vi "Read From String.vi"(8 "error in (no error)":errorcluster, 11 "JSON string":string) -> (0 "error out":errorcluster, 3 "input settings":T1={"PDM clock rate"=51200.0, "decimation factor"=1, "bit clock direction"=enum."In", "logic level"=enum."3.3 V"} {"decimation factor" items=["24"=24, "32"=32, "48"=48, "64"=64, "96"=96, "128"=128]; "PDM clock rate" format="%#_6p"})   [LabVIEW 2022 SP3, in "PDM input cfg file.lvlib"]
uses:
  PDM input cfg file.lvlib
  controls/PDM/PDM input settings.ctl
  <vilib>/PDM Acquisition Toolkit/shared/controls/decimation order.ctl
  controls/bit clock direction.ctl
  <vilib>/PDM Acquisition Toolkit/host/Classes/Session/Controls/Logic Levels.ctl
  controls/PDM/PDM input settings_json.ctl
  <vilib>/PDM Acquisition Toolkit/shared/PDM Shared.lvlib
  <vilib>/PDM Acquisition Toolkit/host/Classes/Session/DecoderSession.lvclass
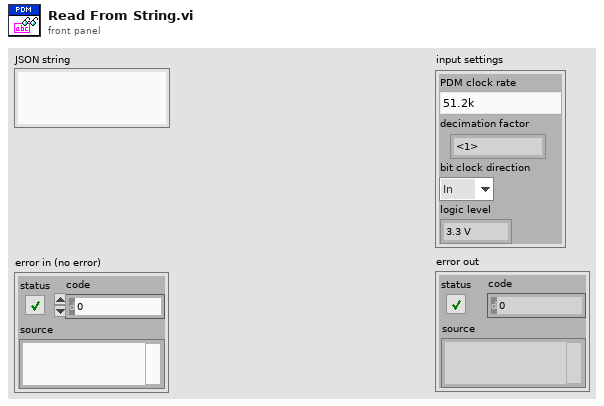
[diagram p1: front panel]
types:
  T1 = typedef "PDM input settings.ctl" = cluster{"PDM clock rate":dbl, "decimation factor":T2, "bit clock direction":T3, "logic level":T4}
  T2 = typedef "PDM Shared.lvlib/decimation order.ctl" = u16
  T3 = typedef "bit clock direction.ctl" = enum32{"In", "Out"}
  T4 = typedef "PDM Acquisition Class Library.lvlib/DecoderSession.lvclass/Logic Levels.ctl" = enum16{"3.3 V", "1.8 V", "1.2 V"}
  T5 = typedef "PDM input settings_json.ctl" = cluster{"PDM clock rate":dbl, "decimation factor":dbl, "bit clock direction":string, "logic level":string}
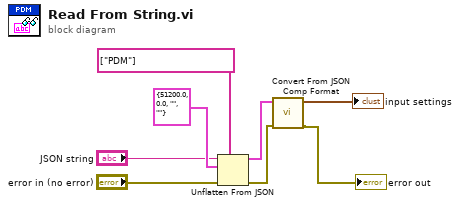
[diagram p0: block diagram]
diagram:
  n1 = Unflatten From JSON(path=string[] ["PDM"], JSON string="JSON string", type and defaults=T5 {"PDM clock rate"=51200.0, "decimation factor"=0.0, "bit clock direction"="", "logic level"=""} ("output settings"), error in (no error)="error in (no error)") -> (value=w2:T5, error out=w7:errorcluster)  [unwired: 3 in]
  n2 = call "Convert From JSON Comp Format.vi"("error in (no error)"=w7, "input settings JSON"=w2) -> ("error out"=→"error out":errorcluster, "input settings"=→"input settings":T1)  [unwired: 8 in]
